vi "ingest.tabular_free.vi"(8 "error in":errorcluster, 11 "TabularIngestStaging in":refnum<class "TabularIngestStaging.lvclass">) -> (0 "error out":errorcluster, 3 "TabularIngestStaging out":refnum<class "TabularIngestStaging.lvclass">)   [LabVIEW 2020, in "TabularIngestStaging.lvclass"]
doc: "Releases the handle and its associated resources."
uses:
  TabularIngestStaging.lvclass
  TabularIngestStaging.lvclass/TabularIngestStaging.ctl
  client.lvlib
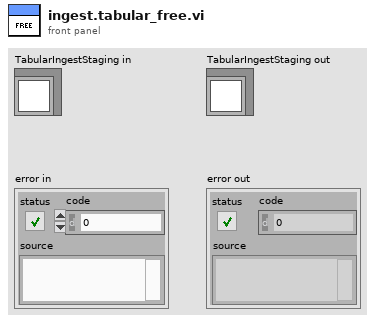
[diagram p1: front panel]
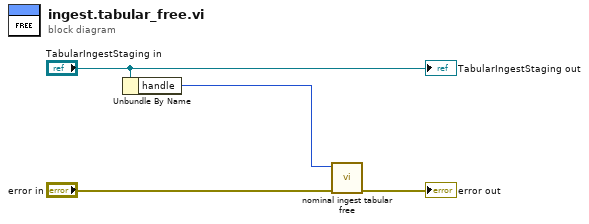
[diagram p0: block diagram]
diagram:
  n1 = Unbundle By Name("TabularIngestStaging in") -> ("handle"=w2:i32)
  n2 = call "nominal ingest tabular free.vi"("error in (no error)"="error in", "staging"=w2) -> ("error out"=→"error out":errorcluster)  [unwired: 8 in, 1 out]
  "TabularIngestStaging out" <- "TabularIngestStaging in"
